vi "Update Select Module Ring.vi"(8 "error in":errorcluster, 11 "Select Module Ring Ref":refnum<vi>) -> (0 "error out":errorcluster, 2 "Active Modules (Array)":string[](array[string]), 3 "New Module Ring Value":i32=-1)   [LabVIEW 2018, in "ModuleInterface.lvlib"]
doc: "Retrieve all currently running cloneable module instances and populate the module selector ring with their names and values.\n_____\nBased on DQMH Project Template 7.0.1.1316."
uses:
  ModuleInterface.lvlib
  Clone Registration/Clone Registration.lvlib
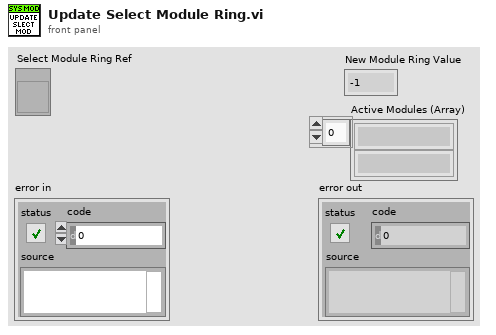
[diagram p1: front panel]
types:
  T1 = typedef "LVStringsAndValuesArrayTypeDef_I32.ctl" = cluster{"String":string, "Value":i32}[]
  T2 = cluster{"Module ID":i32, string, cluster{string, "Module ID":i32}}
  T3 = cluster{"Module ID":i32, string, cluster{string, "Module ID":i32}}[]
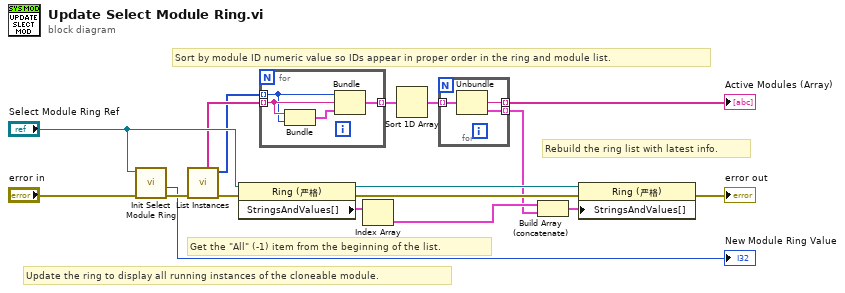
[diagram p0: block diagram]
diagram:
  # "Rebuild the ring list with latest info."
  # "Get the \"All\" (-1) item from the beginning of the list."
  # "Sort by module ID numeric value so IDs appear in proper order in the ring and module list."
  # "Update the ring to display all running instances of the cloneable module."
  n1 = call "Init Select Module Ring.vi"("error in"="error in", "Select Module Ring Ref"="Select Module Ring Ref") -> ("error out"=w13:errorcluster, "Module Ring Value"=→"New Module Ring Value":i32)  [unwired: 7 in, 1 out]
  n2 = call "List Instances.vi"("error in"=w13) -> ("error out"=w17:errorcluster, "Module IDs"=w5:i32[], "Instances Names"=w6:string[])  [unwired: 6 in, 2 out]
  n3 = property on="Property Node" class="Ring (严格)"(reference="Select Module Ring Ref", error in=w17) -> (reference out=w15:refnum<vi>, error out=w16:errorcluster, "StringsAndValues[]"=w8:T1)
  n4 = for {
    tunnel: w6 -> [w20] mode=indexing
    tunnel: w5 -> [w19] mode=indexing
    tunnel: [w21] -> w4 mode=indexing
    n5 = Bundle(w20, "Module ID"=w19) -> (w18:cluster{string, "Module ID":i32})  [unwired: 1 in]
    n6 = Bundle("Module ID"=w19, w20, w18) -> (w21:T2)  [unwired: 1 in]
  }
  n7 = Index Array(array=w8) -> (element=w7:cluster{"String":string, "Value":i32})  [unwired: 1 in]
  n8 = Sort 1D Array(array=w4) -> (sorted array=w3:T3)
  n9 = for {
    tunnel: w3 -> [w24] mode=indexing
    tunnel: [w23] -> w2 mode=indexing
    tunnel: [w22] -> w1 mode=indexing
    n10 = Unbundle(w24) -> (w23:string, w22:cluster{string, "Module ID":i32})  [unwired: 1 out]
  }
  "Active Modules (Array)" <- w2
  n11 = Build Array (concatenate)(w7, w1) -> (w10:cluster{"String":string, "Module ID":i32}[])
  n12 = property on="Property Node" class="Ring (严格)"(reference=w15, error in=w16, "StringsAndValues[]"=w10) -> (error out=→"error out":errorcluster)  [unwired: 1 out]
